vi "MyG#G3SubTempl_GetAttributes.vi"(0 "reference in":refnum<class "MyG#G3SubTempl.lvclass">, 1 "return data":bool=TRUE, 5 "error in (no error)":errorcluster) -> (14 "reference out":refnum<class "MyG#G3SubTempl.lvclass">, 15 "attributes ref":T3, 16 "attributes":T1, 19 "error out":errorcluster)   [LabVIEW 2020, in "MyG#G3SubTempl.lvclass"]
doc: "Returns a reference and if wanted the actual data values of the attributes. This method is used by the subclasses to access parent attributes."
uses:
  MyG#G3SubTempl.lvclass
  C:/Program Files (x86)/National Instruments/LabVIEW 2020/examples/AddQ/G#/CreateDestroy/MyG#G3Templ_class/MyG#G3Templ.lvclass
  ObjectAttributesRef.ctl
  protected/ObjectAttributes.ctl
  MyG#G3Templ_class/protected/ObjectAttributes.ctl
  MyG#G3SubTempl.lvclass/MyG#G3SubTempl.ctl
  MyG#G3Templ_class/MyG#G3Templ.lvclass
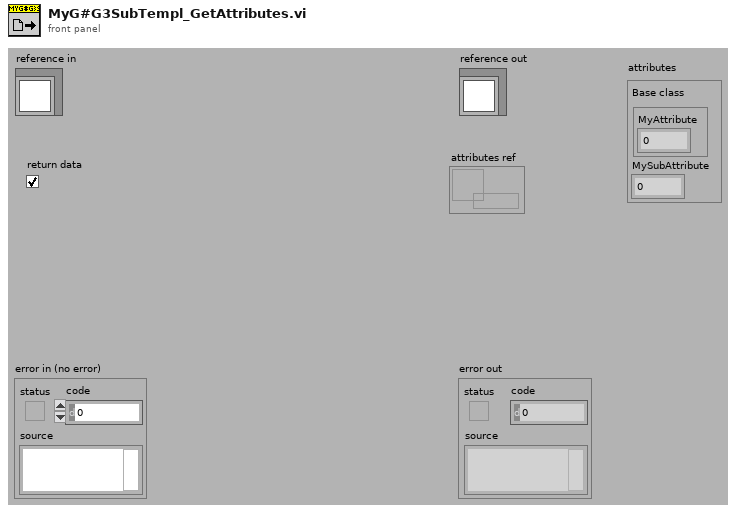
[diagram p1: front panel]
types:
  T1 = typedef "MyG#G3SubTempl.lvclass/ObjectAttributes.ctl" = cluster{"Base class":T2, "MySubAttribute":dbl}
  T2 = typedef "MyG#G3Templ.lvclass/ObjectAttributes.ctl" = cluster{"MyAttribute":dbl}
  T3 = typedef "MyG#G3SubTempl.lvclass/ObjectAttributesRef.ctl" = refnum<data-value>
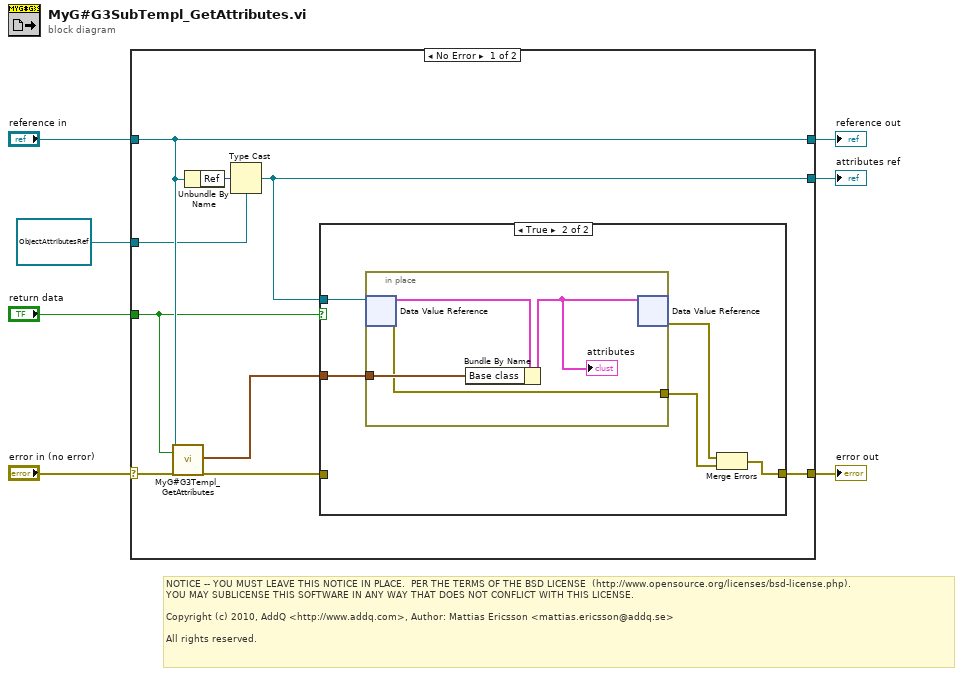
[diagram p0: block diagram]
diagram:
  # "NOTICE -- YOU MUST LEAVE THIS NOTICE IN PLACE.  PER THE TERMS OF THE BSD LICENSE  (http://www.opensource.org/licenses/bsd-license.php).\nYOU MAY SUBLICENSE THIS SOFTWARE IN ANY WAY THAT DOES NOT CONFLICT WITH THIS LICENSE.\n\nCopyright (c) 2010, AddQ <http://www.addq.com>, Author: Mattias Ericsson <mattias.ericsson@addq.se>\n\nAll rights reserved."
  n1 = case shown="No Error" "error in (no error)" {
    selector: "error in (no error)" -> [w15 w29]
    tunnel: [w16 w29] -> w6
    tunnel: [w13 w28] -> w4
    tunnel: "reference in" -> [w13 w28]
    tunnel: [w9 w27] -> w3
    tunnel: "return data" -> [w12 _]
    tunnel: T3 refnum ("attributes ref") -> [w8 w27]
    frame No Error {
      n2 = call "MyG#G3Templ_GetAttributes.vi"("reference in"=w13, "return data"=w12, "error in (no error)"=w15) -> ("attributes"=w11:T2, "error out"=w14:errorcluster)  [unwired: 13 in, 2 out]
      n3 = Unbundle By Name(w13) -> ("Ref"=w10:u32)
      n4 = Type Cast(type=w8, x=w10) -> (*(type *) &x=w9:T3)
      n5 = case shown="True" w12 {
        tunnel: w9 -> [_ w22]
        tunnel: w14 -> [w17 _]
        tunnel: [w17 w19] -> w16
        tunnel: w11 -> [_ w18]
        frame False {
        }
        frame True {
          n6 = in-place {
            in-place-border: [w23] -> w21
            in-place-border: w18 -> [w24]
            n7 = in-place-dvr #1(w22) -> (w26:T1, w23:errorcluster)
            n8 = Bundle By Name(cluster=w26, "Base class"=w24) -> (w25:T1)
            "attributes" <- w25
            n9 = in-place-dvr #1(w25) -> (w20:errorcluster)  [unwired: 1 out]
          }
          n10 = Merge Errors(w20, w21) -> (w19:errorcluster)
        }
      }
    }
    frame Error {
    }
  }
  "error out" <- w6
  "reference out" <- w4
  "attributes ref" <- w3
